vi "Generate grid trap cluster (SubVI).vi"(6 "output cluster 3":T2, 8 "Coordinate mapping \n(IMAQ to SLM)":T1={"sX"=-256.0, "sY"=-256.0, "sZ"=0.0, "cX"=0.5, "cY"=0.5, "cZ"=1.0}, 9 "Grid spacing":i32, 10 "Spots y":i32, 11 "Spots x":i32) -> (3 "output cluster 2":T2)   [LabVIEW 2011]
uses:
  Trap cluster.ctl
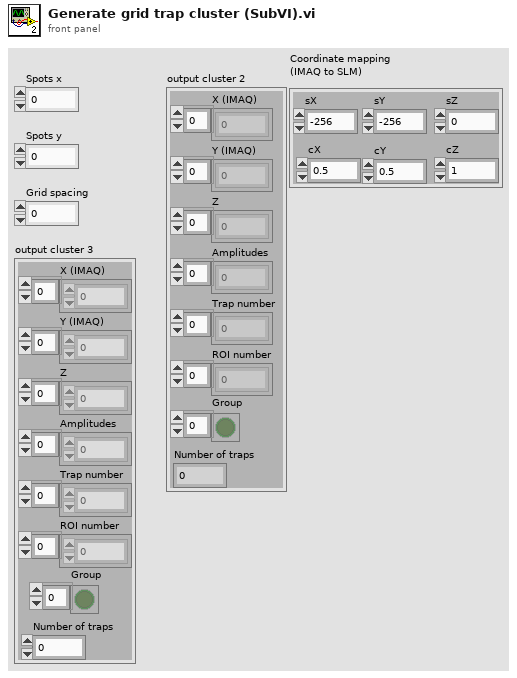
[diagram p1: front panel]
types:
  T1 = cluster{"sX":dbl, "sY":dbl, "sZ":dbl, "cX":dbl, "cY":dbl, "cZ":dbl}
  T2 = typedef "Trap cluster.ctl" = cluster{"X (IMAQ)":dbl[], "Y (IMAQ)":dbl[], "Z":dbl[], "Amplitudes":dbl[], "Trap number":i32[], "ROI number":i32[], "Number of traps":i32, "Group":bool[]}
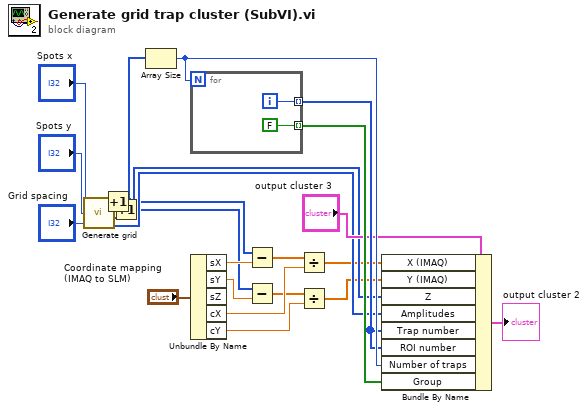
[diagram p0: block diagram]
diagram:
  n1 = call "Generate grid.vi"("Spots x"="Spots x", "Spots y"="Spots y", "Grid spacing"="Grid spacing") -> ("X"=w6:i32[], "Y"=w5:i32[], "Z"=w17:i32[], "A"=w18:i32[])
  n2 = Increment(x=w6) -> (x+1=w2:i32[])
  n3 = Increment(x=w5) -> (x+1=w1:i32[])
  n4 = Array Size(array=w2) -> (size(s)=w22:i32)
  n5 = for {
    N: w22 -> [_]
    tunnel: [w25] -> w21 mode=indexing
    tunnel: [FALSE ("Boolean")] -> w23 mode=indexing
    i -> [w25]
  }
  n6 = Unbundle By Name("Coordinate mapping \n(IMAQ to SLM)") -> ("sX"=w13:dbl, "sY"=w11:dbl, "cX"=w14:dbl, "cY"=w12:dbl)  [unwired: 1 out]
  n7 = Subtract(x=w2, y=w13) -> (x-y=w8:dbl[])
  n8 = Subtract(x=w1, y=w11) -> (x-y=w4:dbl[])
  n9 = Divide(x=w8, y=w14) -> (x/y=w7:dbl[])
  n10 = Divide(x=w4, y=w12) -> (x/y=w3:dbl[])
  n11 = Bundle By Name(cluster="output cluster 3", "X (IMAQ)"=w7, "Y (IMAQ)"=w3, "Z"=w17, "Amplitudes"=w18, "Trap number"=w21, "ROI number"=w21, "Number of traps"=w22, "Group"=w23) -> (→"output cluster 2":T2)
